vi "Coerce Frequency (Fs, N).vi"(9 "Npts":i32, 10 "Sampling rate (Hz)":dbl, 11 "Frequency (kHz)":dbl[](array[numeric])) -> (1 "Npts":i32, 2 "Sampling rate (Hz)":dbl, 3 "Coerced Frequency (kHz)":dbl[](array[numeric]))   [LabVIEW 2015]
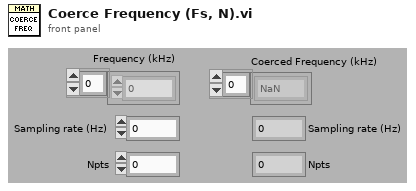
[diagram p1: front panel]
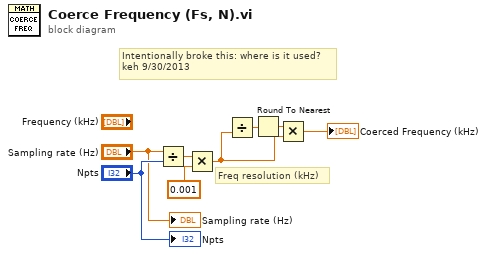
[diagram p0: block diagram]
diagram:
  # "Intentionally broke this: where is it used?\nkeh 9/30/2013"
  # "Freq resolution (kHz)"
  n1 = Divide(x="Sampling rate (Hz)", y="Npts") -> (x/y=w8:dbl)
  n2 = Multiply(x=w8, y=0.001) -> (x*y=w5:dbl)
  n3 = Divide(y=w5) -> (x/y=w7:dbl)  [unwired: 1 in]
  n4 = Round To Nearest(number=w7) -> (nearest integer value=w6:dbl)
  n5 = Multiply(x=w6, y=w5) -> (x*y=→"Coerced Frequency (kHz)":dbl)
  "Sampling rate (Hz)" <- "Sampling rate (Hz)"
  "Npts" <- "Npts"
